vi "Demo Temperature Read.vi"() -> (0 "Measured Temperature (degC)":dbl format="%.2f")   [LabVIEW 2020]
doc: "This subVI simulates taking one single temperature measurement. Every time it is called, you will get a differenttemperature value. It generates one value at a time from a pre-stored array of values."
panel:
  # "This subVI simulates taking one \nsingle temperature measurement.\nEvery time it is called, you will get a different\ntemperature value"
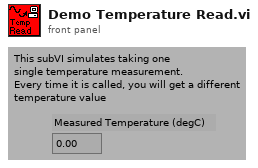
[diagram p1: front panel]
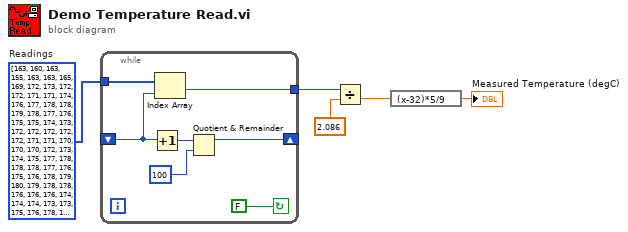
[diagram p0: block diagram]
diagram:
  w3 = i32[] [163, 160, 163, 155, 163, 163, 165, 169, 172, 173, 172, 172, 171, 171, 174, 176, 177, 178, 178, 179, 178, 177, 176, 175, 175, 174, 173, 172, 172, 172, 172, 172, 171, 171, 170, 170, 170, 172, 173, 174, 175, 177, 178, 178, 178, 177, 176, 175, 176, 178, 179, 180, 179, 178, 178, 176, 176, 176, 174, 174, 174, 173, 173, 175, 176, 178, 178, 177, 176, 175, 175, 174, 174, 173, 173, 172, 172, 171, 171, 170, 170, 170, 170, 170, 170, 170, 169, 166, 167, 169, 170, 169, 168, 168, 168, 168, 167, 167, 167, 167]  # Readings
  n1 = while {
    tunnel: w3 -> [w7]
    tunnel: [w8] -> w5
    shift-left: _ -> [w12]
    shift-right: [w9] -> _
    stop <- FALSE continue-if-true
    n2 = Increment(x=w12) -> (x+1=w11:i32)
    n3 = Index Array(array=w7, index=w12) -> (element=w8:i32)
    n4 = Quotient & Remainder(x=w11, y=100) -> (x-y*floor(x/y)=w9:i32)  [unwired: 1 out]
  }
  n5 = Divide(x=w5, y=2.086) -> (x/y=w2:dbl)
  n6 = expression code="(x-32)*5/9"(w2) -> (→"Measured Temperature (degC)":dbl)
